vi "Create New VI or CTL On Disk.vi"(7 "VI Description":string, 8 "error in":errorcluster, 9 "Application Instance Ref":refnum<vi>, 10 "Selected Template VI or CTL name (including file extension)":string, 11 "Filepath of VI or CTL to be created":path) -> (0 "error out":errorcluster, 3 "Reference of newly created VI":refnum<vi>)   [LabVIEW 2022 SP3]
doc: "This VI creates a new VI or CTL on disk as a \"Save as...\" copy of a template VI or CTL.\n\nThis VI doesn't insert the newly created VI into a project, lvlib, or lvclass. That is done in another VI."
panel:
  # "Development\ncontrols/indicators useful for development and testing, but which are not outputs of the VI"
  # "Input\nInputs to the VI"
  # "Output\nOutputs of the VI"
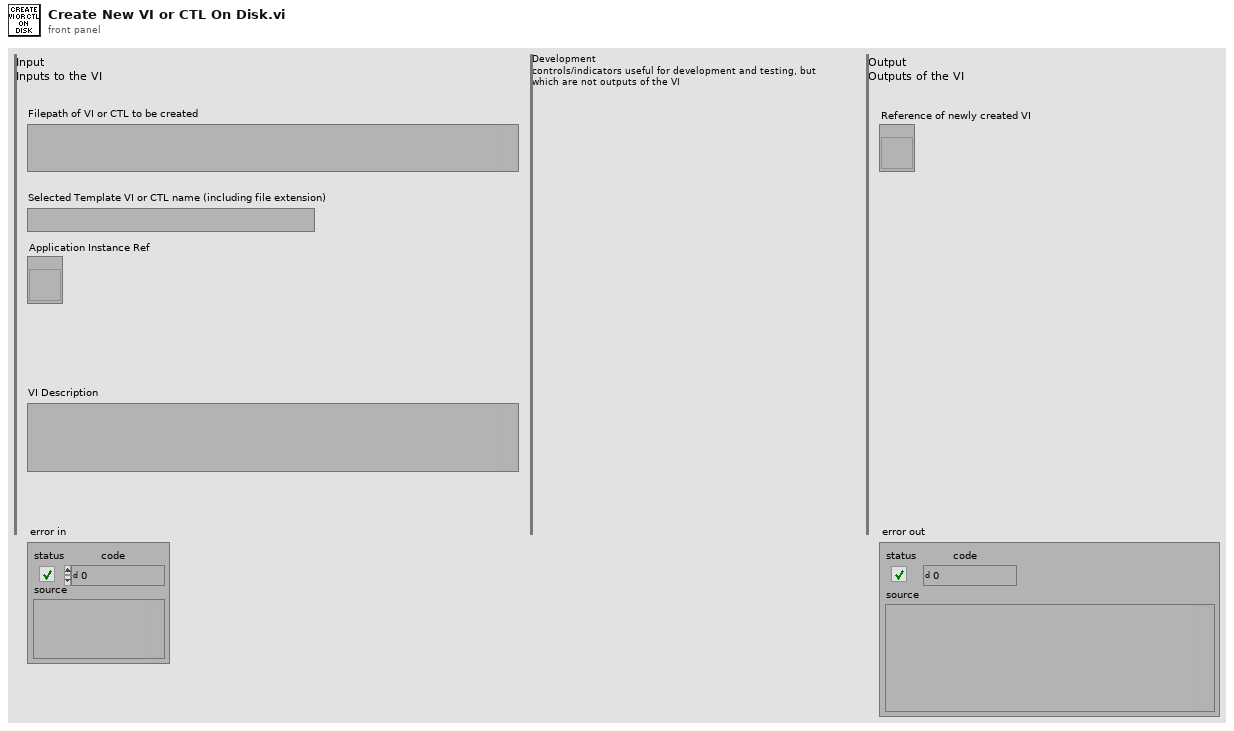
[diagram p1: front panel]
types:
  T1 = enum32{"invalid VI type", "Standard VI", "Control VI", "Global VI", "Polymorphic VI", "Configuration VI", "SubSystem", "Facade VI", "Method VI", "Statechart Diagram VI"}
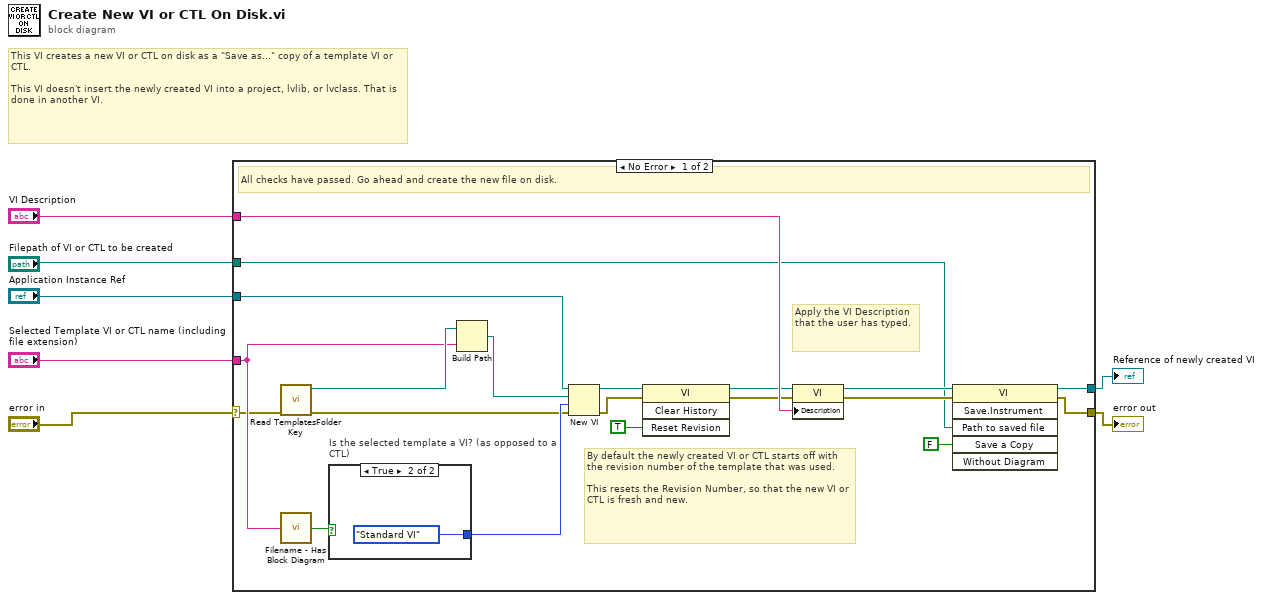
[diagram p0: block diagram]
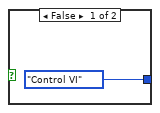
[diagram p2: hidden frame]
diagram:
  # "This VI creates a new VI or CTL on disk as a \"Save as...\" copy of a template VI or CTL.\n\nThis VI doesn't insert the newly created VI into a project, lvlib, or lvclass. That is done in another VI."
  n1 = case shown="No Error" "error in" {
    selector: "error in" -> [w9 w30]
    tunnel: [w12 w30] -> w6
    tunnel: "Selected Template VI or CTL name (including file extension)" -> [w20 _]
    tunnel: [w11 _] -> w4
    tunnel: "VI Description" -> [w17 _]
    tunnel: "Filepath of VI or CTL to be created" -> [w10 _]
    tunnel: "Application Instance Ref" -> [w8 _]
    frame No Error {
      # "Apply the VI Description that the user has typed."
      # "By default the newly created VI or CTL starts off with the revision number of the template that was used.\n\nThis resets the Revision Number, so that the new VI or CTL is fresh and new."
      # "All checks have passed. Go ahead and create the new file on disk."
      n2 = call "Read TemplatesFolder Key.vi"("Error In"=w9) -> ("Error Out"=w21:errorcluster, "Templates Folder Path"=w22:path)  [unwired: 9 in]
      n3 = call "Filename - Has Block Diagram.vi"("Filename (including file extension)"=w20) -> ("Has Block Diagram?"=w19:bool)
      n4 = case "Is the selected template a VI? (as opposed to a CTL)" shown="True" w19 {
        tunnel: [T1."Control VI" ("vi type (standard vi)") T1."Standard VI" ("vi type (standard vi)")] -> w26
        frame False {
        }
        frame True {
        }
      }
      n5 = Build Path(base path=w22, name or relative path=w20) -> (appended path=w27:path)
      n6 = New VI(8:w21, 9:w26, 10:w27, 11:w8) -> (0:w24:errorcluster, 3:w25:refnum<vi>)  [unwired: 3 in]
      n7 = invoke class="VI" method="Clear History"(reference=w25, error in=w24, "Reset Revision"=TRUE) -> (reference out=w15:refnum<vi>, error out=w16:errorcluster)  [unwired: 1 in, 2 out]
      n8 = property class="VI"(reference=w15, error in=w16, "Description"=w17) -> (reference out=w13:refnum<vi>, error out=w14:errorcluster)
      n9 = invoke class="VI" method="Save.Instrument"(reference=w13, error in=w14, "Path to saved file"=w10, "Save a Copy"=FALSE) -> (reference out=w11:refnum<vi>, error out=w12:errorcluster)  [unwired: 2 in, 4 out]
    }
    frame Error {
      # "Do nothing. The error message will be handled later, downstream"
      # "One or more checks failed."
    }
  }
  "error out" <- w6
  "Reference of newly created VI" <- w4
